vi "State Enter Core.vi"(8 "error in (no error)":errorcluster, 11 "B Context State in":refnum<class "B Context State.lvclass">) -> (0 "error out":errorcluster, 3 "B Context State out":refnum<class "B Context State.lvclass">)   [LabVIEW 2021, in "Context Actor.lvlib" / "B Context State.lvclass"]
uses:
  B Context State.lvclass
  B Context State.lvclass/B Context State.ctl
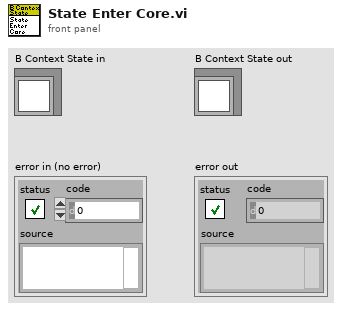
[diagram p1: front panel]
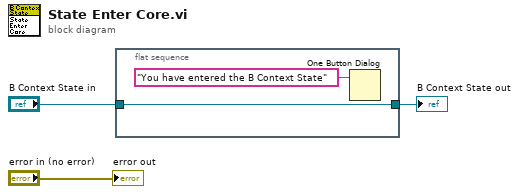
[diagram p0: block diagram]
diagram:
  n1 = flat-sequence {
    tunnel: [w4] -> w1
    tunnel: "B Context State in" -> [w4]
    frame #0 {
      n2 = One Button Dialog(message="You have entered the B Context State") -> ()  [unwired: 1 in, 1 out]
    }
  }
  "error out" <- "error in (no error)"
  "B Context State out" <- w1
